vi "lua_close.vi"(8 "error in (no error)":errorcluster, 11 "lua_state_p":u64) -> (0 "error out":errorcluster)   [LabVIEW 2020, in "lua.dll.lvlib"]
uses:
  lua.dll.lvlib
  lua54.dll
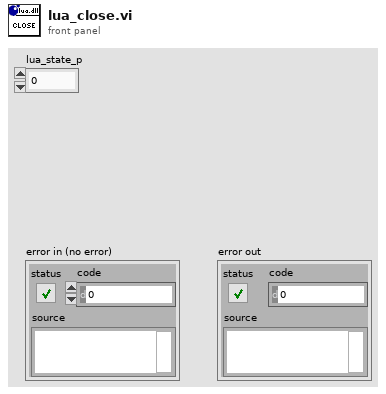
[diagram p1: front panel]
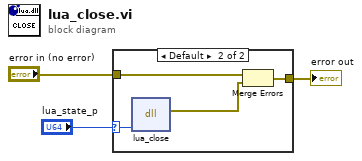
[diagram p0: block diagram]
diagram:
  n1 = case shown="Default" "lua_state_p" {
    selector: "lua_state_p" -> [_ w8]
    tunnel: [w4 w5] -> w3
    tunnel: "error in (no error)" -> [w4 w6]
    frame 0 {
    }
    frame Default {
      n2 = dll-call lib="C:/Users/Nicholas Folse/Documents/workspace/github-tauterra.llc/Lua for LabVIEW/lib/lua.dll/lua54**.*" fn="lua_close"("lua_state_p"=w8) -> (error out=w7:errorcluster)  [unwired: 5 in, 1 out]
      n3 = Merge Errors(w6, w7) -> (w5:errorcluster)
    }
  }
  "error out" <- w3
